vi "Format Type String.vi"(8 "error in (no error)":errorcluster, 10 "Pre-Name":string, 11 "Data Type":variant) -> (0 "error out":errorcluster, 2 "Type Name":string)   [LabVIEW 2020, in "VariantExtensions.lvlib"]
doc: "格式类型字符串"
uses:
  VariantExtensions.lvlib
  <vilib>/Utility/Data Type/NI_Data Type.lvlib
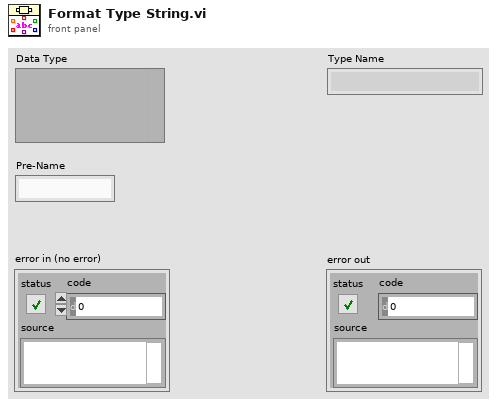
[diagram p1: front panel]
types:
  T1 = typedef "NI_Data Type.lvlib/Data Type.ctl" = enum8{"Invalid Type", "Void", "I8", "I16", "I32", "I64", "U8", "U16", "U32", "U64", "Single Float", "Double Float", "Extended Float", "Single Complex", "Double Complex", "Extended Complex", "Enum U8", "Enum U16", "Enum U32", "Enum U64", "Single Float With Unit", "Double Float With Unit", "Extended Float With Unit", "Single Complex with Unit", "Double Complex with Unit", "Extended Complex with Unit", "Boolean", "String", "Path", "Picture", "Tag", "Array", "Cluster", "Variant", "LV Variant", "Waveform", "Timestamp", "Digital Waveform", "Digital Data", "ExpressData", "Refnum", "External Data", "VI", "Poly VI", "LabVIEW Class Instance", "Fixed Point", "Set Collection", "Map Collection"}
  T2 = typedef "NI_Data Type.lvlib/Type Definition Info.ctl" = cluster{"Name":string, "Timestamp":u32}
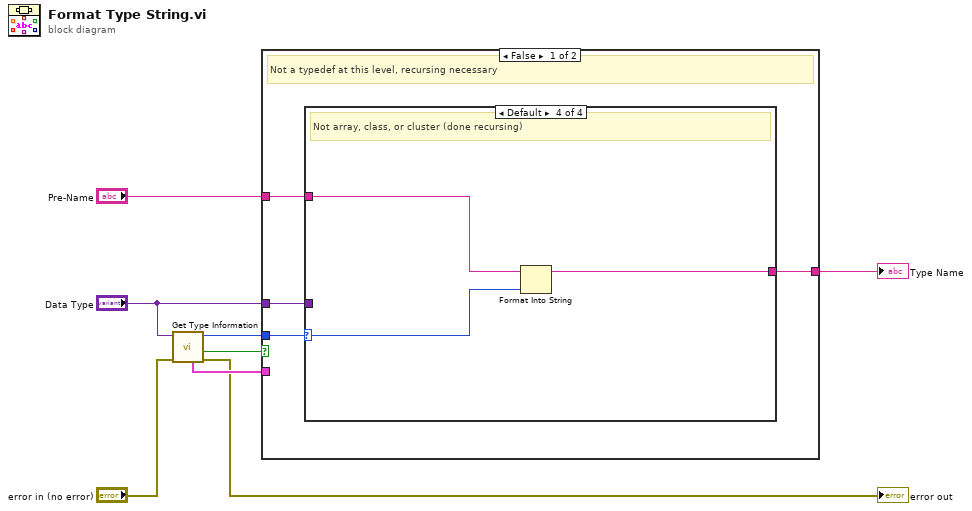
[diagram p0: block diagram]
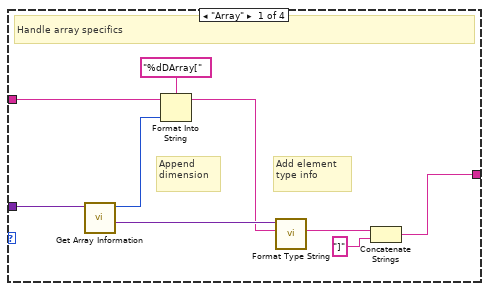
[diagram p2: hidden frame]
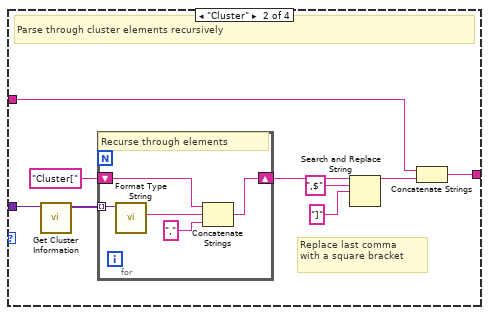
[diagram p3: hidden frame]
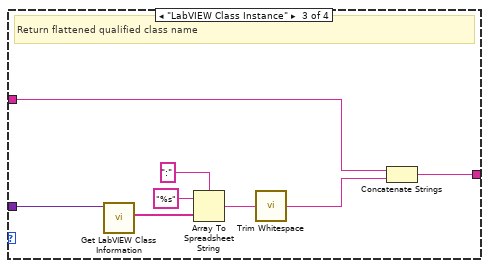
[diagram p4: hidden frame]
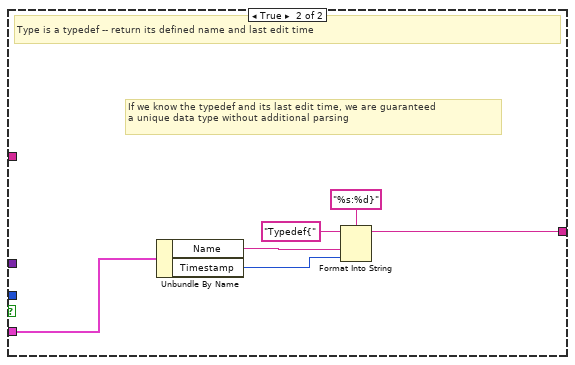
[diagram p5: hidden frame]
diagram:
  n1 = call <vilib>:"Get Type Information.vi"("error in (no error)"="error in (no error)", "variant"="Data Type") -> ("error out"=→"error out":errorcluster, "type definition"=w5:bool, "type"=w4:T1, "type definition info"=w6:T2)  [unwired: 5 in, 1 out]
  n2 = case shown="False" w5 {
    tunnel: [w12 w48] -> w8
    tunnel: "Data Type" -> [w11 _]
    tunnel: "Pre-Name" -> [w10 _]
    tunnel: w4 -> [w9 _]
    tunnel: w6 -> [_ w52]
    frame False {
      # "Not a typedef at this level, recursing necessary"
      n3 = case shown="Default" w9 {
        selector: w9 -> [_ _ _ w46]
        tunnel: [w15 w27 w37 w44] -> w12
        tunnel: w11 -> [w21 w30 w43 _]
        tunnel: w10 -> [w20 w28 w36 w45]
        frame "Array" {
          # "Append\ndimension"
          # "Add element\ntype info"
          # "Handle array specifics"
          n4 = call <vilib>:"Get Array Information.vi"("variant"=w21) -> ("array element data type"=w19:variant, "number of dimensions"=w17:i32)  [unwired: 7 in, 2 out]
          n5 = Format Into String(format string="%dDArray[", initial string=w20, w17) -> (resulting string=w13:string)  [unwired: 1 in, 1 out]
          n6 = call "Format Type String.vi"("Pre-Name"=w13, "Data Type"=w19) -> ("Type Name"=w18:string)  [unwired: 8 in, 1 out]
          n7 = Concatenate Strings(w18, "]" ("string")) -> (w15:string)
        }
        frame "Cluster" {
          # "Replace last comma\nwith a square bracket"
          # "Parse through cluster elements recursively"
          n8 = call <vilib>:"Get Cluster Information.vi"("variant"=w30) -> ("cluster elements"=w29:variant[])  [unwired: 9 in, 1 out]
          n9 = for {
            tunnel: w29 -> [w35] mode=indexing
            shift-right: [w33] -> w25
            shift-left: "Cluster[" ("string") -> [w31]
            # "Recurse through elements"
            n10 = call "Format Type String.vi"("Data Type"=w35) -> ("Type Name"=w34:string)  [unwired: 9 in, 1 out]
            n11 = Concatenate Strings(w31, w34, "," ("string")) -> (w33:string)
          }
          n12 = Search and Replace String(input string=w25, search string=",$", replace string="]" ("string")) -> (result string=w22:string)  [unwired: 5 in, 3 out]
          n13 = Concatenate Strings(w28, w22) -> (w27:string)
        }
        frame "LabVIEW Class Instance" {
          # "Return flattened qualified class name"
          n14 = call <vilib>:"Get LabVIEW Class Information.vi"("variant"=w43) -> ("qualified LabVIEW class name"=w42:string[])  [unwired: 8 in, 2 out]
          n15 = Array To Spreadsheet String(delimiter (Tab)=":", array=w42, 3:"%s" ("format string")) -> (spreadsheet string=w39:string)
          n16 = call <vilib>:"Trim Whitespace.vi"("string"=w39) -> ("trimmed string"=w38:string)  [unwired: 1 in]
          n17 = Concatenate Strings(w36, w38) -> (w37:string)
        }
        frame Default {
          # "Not array, class, or cluster (done recursing)"
          n18 = Format Into String(initial string=w45, w46) -> (resulting string=w44:string)  [unwired: 2 in, 1 out]
        }
      }
    }
    frame True {
      # "If we know the typedef and its last edit time, we are guaranteed\na unique data type without additional parsing"
      # "Type is a typedef -- return its defined name and last edit time"
      n19 = Unbundle By Name(w52) -> ("Name"=w51:string, "Timestamp"=w47:u32)
      n20 = Format Into String(format string="%s:%d}", initial string="Typedef{", w51, w47) -> (resulting string=w48:string)  [unwired: 1 in, 1 out]
    }
  }
  "Type Name" <- w8
